vi "SS2 Live_Globals.vi"() -> ()   [LabVIEW 2019]
panel:
  in  "Admin":bool
  in  "Settings Window Refnum":refnum<vi>
  in  "SS2 Live Version":string
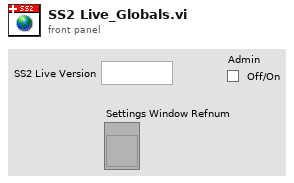
[diagram p1: front panel]
diagram:
